vi "Thigh Angle PCA v4.vi"(7 "Num Data Point":i32=2000, 8 "error in (no error)":errorcluster, 10 "byte count":u32, 11 "VISA resource name":refnum<visa-resource-name>) -> (0 "error out":errorcluster, 1 "w_pitch":dbl, 2 "w_roll":dbl, 3 "weights":dbl[][](array[numeric]))   [LabVIEW 2018]
uses:
  <vilib>/Platform/TimedLoop/XDataNode/timing_clust.ctl
  <vilib>/Platform/TimedLoop/XDataNode/nitl_modes.ctl
  <vilib>/Platform/TimedLoop/XDataNode/wakeup.ctl
  <vilib>/addons/Time Series Analysis/Statistical Analysis.llb/TSA Principal Component Analysis (Array).vi
  <vilib>/platform/TimedLoop/XDataNode/XDataNode.xnode
  <vilib>/Platform/TimedLoop/XDataNode/XDNodeRunTimeDep.lvlib
  <vilib>/addons/_Advanced Signal Processing/NI_AdvSigProcTSA.lvlib
panel:
  out "size(s)":i32[](array[numeric])
  out "Array":dbl[][](array[numeric])
  out "Waveform Chart":T1(graph)
  out "Period [uS]":u32
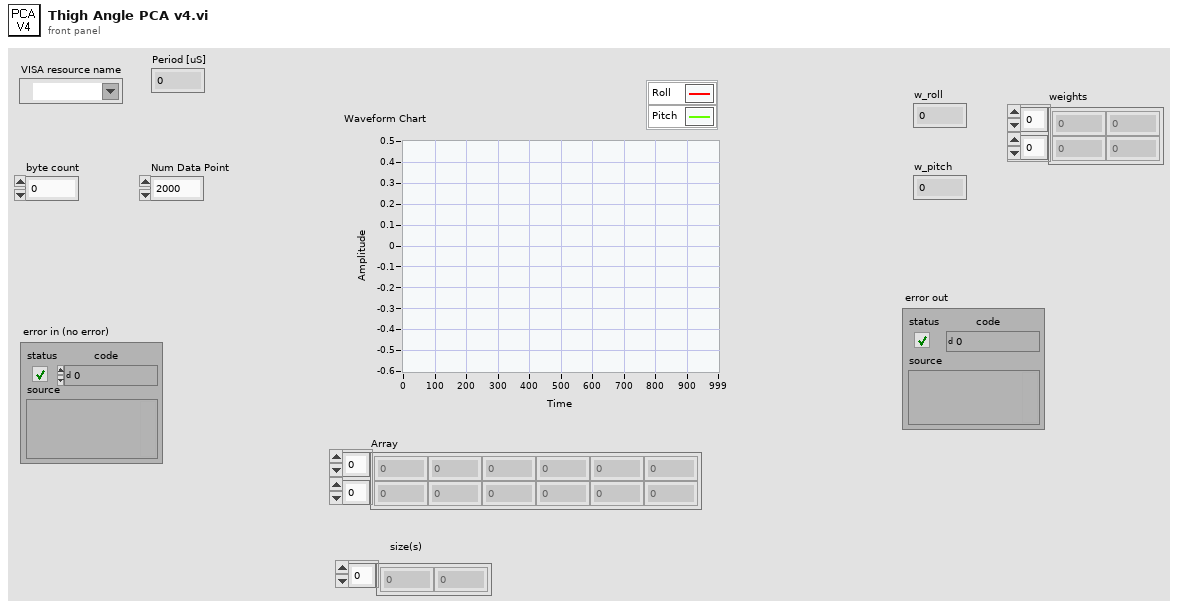
[diagram p1: front panel]
types:
  T1 = cluster{"Roll Angle [rad]":dbl, "Pitch Angle [rad]":dbl}
  T2 = typedef "XDNodeRunTimeDep.lvlib/timing_clust.ctl" = cluster{"Expected End [f-1]":u64, "Actual End [f-1]":u64, "Finished Late? [f-1]":bool, "Expected End [i-1]":u64, "Actual End [i-1]":u64, "Finished Late? [i-1]":bool, "Expected Start [i]":u64, "Actual Start [i]":u64, "Expected Start [f]":u64, "Actual Start [f]":u64, "Source Name":string, "Structure Name":string, "Period":i64, "Deadline":i64, "Offset":i64, "Start":i64, "Priority":i32, "Timeout":i32, "Mode":T3, "Wakeup Reason":T4, "Error":errorcluster, "Source Type":string, "Secondary Source Type":string, "Global End Time":u64, "Global Start Time":u64, "Frame Duration":u64, "Iteration Duration":u64, "Assigned CPU":i32, "I/O Scan Engine Mode":u32}
  T3 = typedef "XDNodeRunTimeDep.lvlib/nitl_modes.ctl" = enum32{"No Change", "Process missed periods, maintain original phase", "Discard missed periods, maintain original phase", "Process missed periods, ignore original phase", "Discard missed periods, ignore original phase"}
  T4 = typedef "XDNodeRunTimeDep.lvlib/wakeup.ctl" = enum32{"Normal", "Aborted", "Asynchronous wakeup", "Timing source error", "Timed loop error", "Timeout"}
  T5 = typedef "NI_Matrix.lvlib/RealMatrix.ctl" = dbl[][]
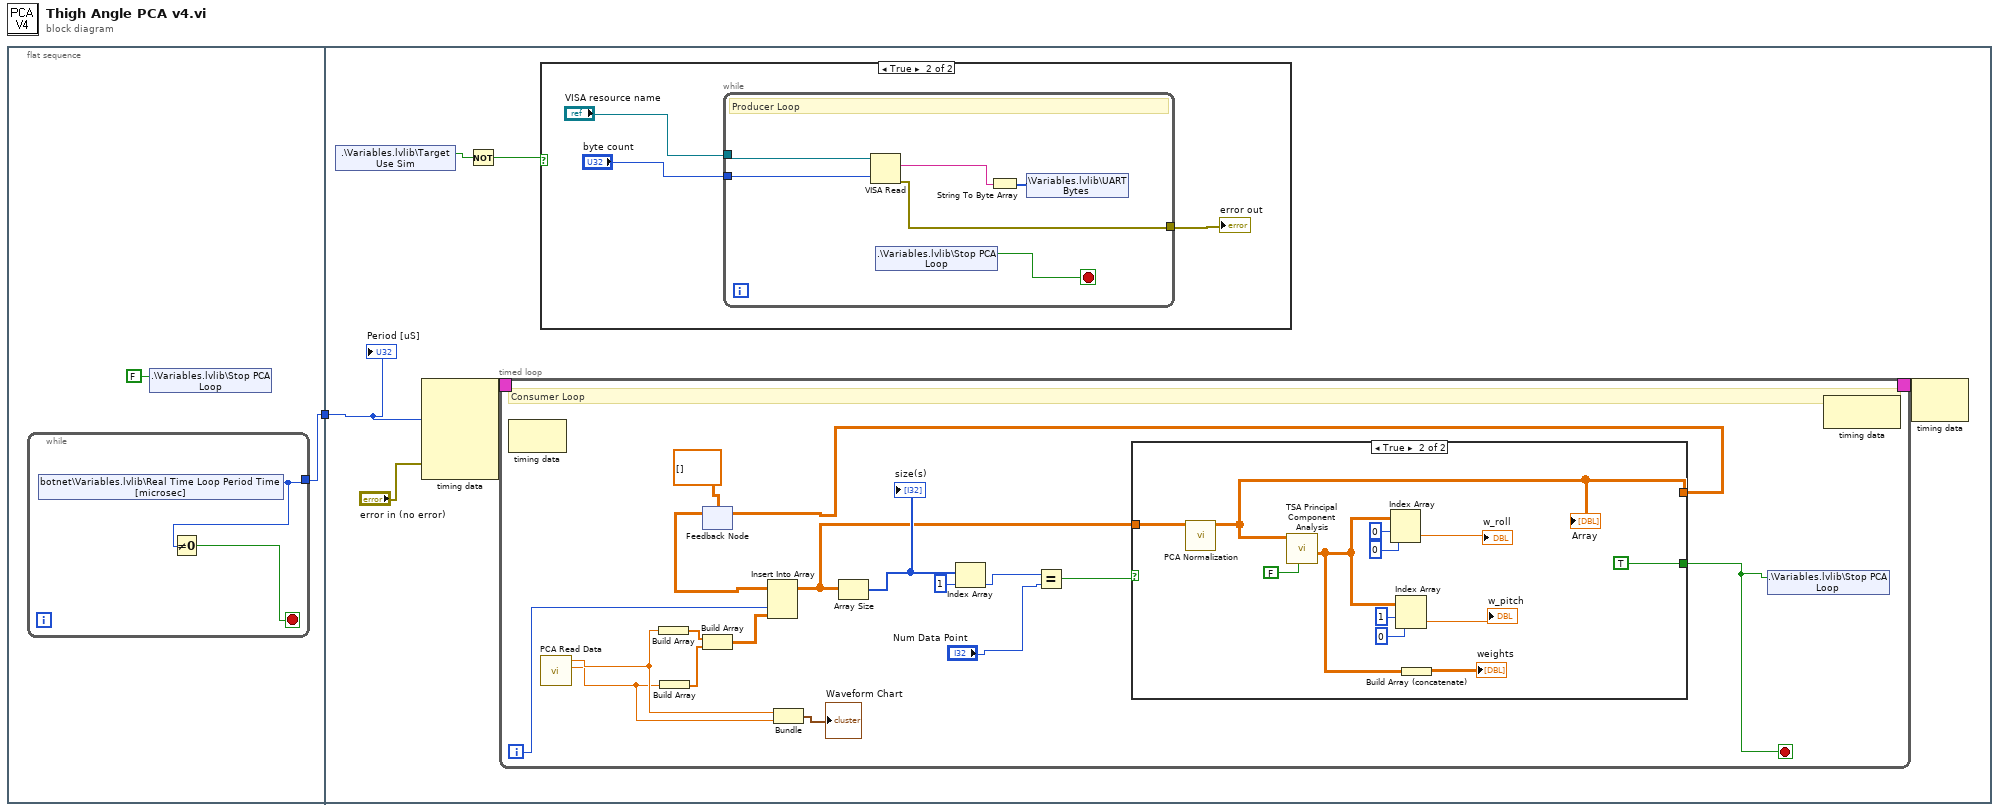
[diagram p0: block diagram]
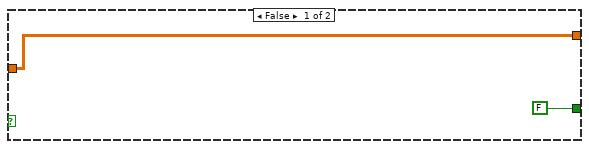
[diagram p3: hidden frame]
diagram:
  n1 = flat-sequence {
    tunnel: [w2] -> w1
    tunnel: w1 -> [w8]
    frame #0 {
      n2 = while {
        tunnel: [w4] -> w2
        stop <- w5 stop-if-true
        n3 = shared-variable "botnet\\Variables.lvlib\\Real Time Loop Period Time [microsec]"() -> (w4:u32)  [unwired: 1 in, 1 out]
        n4 = Not Equal To 0?(x=w4) -> (x != 0?=w5:bool)
      }
      n5 = shared-variable ".\\Variables.lvlib\\Stop PCA Loop"(FALSE ("Stop PCA Loop")) -> ()  [unwired: 1 in, 1 out]
    }
    frame #1 {
      n6 = shared-variable ".\\Variables.lvlib\\Target Use Sim"() -> (w7:bool)  [unwired: 1 in, 1 out]
      n7 = node-c288(w8, "error in (no error)") -> (w11:T2)  [unwired: 3 in]
      n8 = Not(x=w7) -> (.not. x?=w6:bool)
      n9 = timed-loop {
        timing: w11 -> [_]
        timing-out: [_] -> w10
        i -> [w23]
        stop <- w37 stop-if-true
        # "Consumer Loop"
        n10 = node-c288() -> ()  [unwired: 1 in, 1 out]
        n11 = call "PCA Read Data.vi"() -> ("Pitch"=w21:dbl, "Roll"=w22:dbl)  [unwired: 10 in]
        n12 = Build Array(w22) -> (w26:dbl[])
        n13 = Build Array(w21) -> (w25:dbl[])
        n14 = feedback #1(dbl[][] []) -> (w35:dbl[][])
        n15 = Build Array "Build Array"(w26, w25) -> (w33:dbl[][])
        n16 = Insert Into Array "Insert Into Array"(array=w35, index (col)=w23, new element=w33) -> (w27:dbl[][])  [unwired: 1 in]
        n17 = Bundle("Roll"=w22, "Pitch"=w21) -> (→"Waveform Chart":cluster{"Roll":dbl, "Pitch":dbl})  [unwired: 1 in]
        n18 = Array Size(array=w27) -> (size(s)=w32:i32[])
        "size(s)" <- w32
        n19 = Index Array(array=w32, index=1) -> (element=w30:i32)
        n20 = Equal?(x=w30, y="Num Data Point") -> (x = y?=w28:bool)
        n21 = case shown="True" w28 {
          tunnel: w27 -> [w41 w43]
          tunnel: [w41 w42] -> w24
          tunnel: [FALSE TRUE] -> w37
          frame False {
          }
          frame True {
            n22 = call "PCA Normalization.vi"("Original Array"=w43) -> ("Zero Mean Array"=w42:dbl[][])  [unwired: 10 in]
            "Array" <- w42
            n23 = call-poly <vilib>:"TSA Principal Component Analysis.vi"("unified? (F)"=FALSE, "Xt"=w42) -> ("weights"=w44:dbl[][])  [unwired: 6 in, 3 out]
            n24 = Index Array(array=w44, index (row)=0, index (col)=0 ("disabled index (col)")) -> (element=→"w_roll":dbl)
            n25 = Index Array(array=w44, index (row)=1, index (col)=0 ("disabled index (col)")) -> (element=→"w_pitch":dbl)
            n26 = Build Array (concatenate)(w44) -> (→"weights":T5)
          }
        }
        n27 = feedback-in #1(w24) -> ()
        n28 = shared-variable ".\\Variables.lvlib\\Stop PCA Loop"(w37) -> ()  [unwired: 1 in, 1 out]
        n29 = node-c288() -> ()  [unwired: 1 in, 1 out]
      }
      n30 = case shown="True" w6 {
        frame False {
        }
        frame True {
          n31 = while {
            tunnel: "byte count" -> [w20]
            tunnel: [w19] -> w13
            tunnel: "VISA resource name" -> [w15]
            stop <- w16 stop-if-true
            # "Producer Loop"
            n32 = VISA Read(VISA resource name=w15, byte count=w20) -> (read buffer=w18:string, error out=w19:errorcluster)  [unwired: 1 in, 2 out]
            n33 = shared-variable ".\\Variables.lvlib\\Stop PCA Loop"() -> (w16:bool)  [unwired: 1 in, 1 out]
            n34 = String To Byte Array(string=w18) -> (unsigned byte array=w17:u8[])
            n35 = shared-variable ".\\Variables.lvlib\\UART Bytes"(w17) -> ()  [unwired: 1 in, 1 out]
          }
          "error out" <- w13
        }
      }
      n36 = node-c288(w10) -> ()  [unwired: 1 out]
      "Period [uS]" <- w8
    }
  }
